vi "Archive Mixed Mode State.vi"(8 "error in":errorcluster, 11 "MixedModeStates":T1) -> (0 "error out":errorcluster, 2 "string":string)   [LabVIEW 2009]
uses:
  Mixed Mode States.ctl
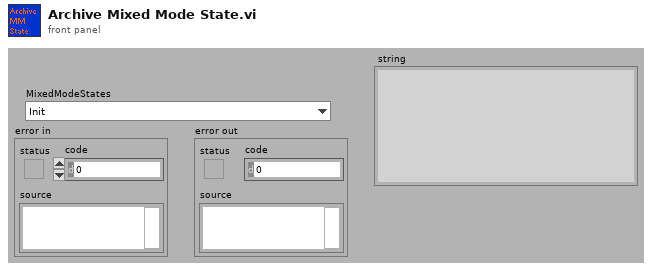
[diagram p1: front panel]
types:
  T1 = typedef "Mixed Mode States.ctl" = enum16{"Init", "Idle", "Start Initial Ramp", "Run Initial Ramp", "Start Iterative Stage", "Convergence Check", "Update Stiffness Jacobian", "Update Command", "Start Iterative Ramp", "Run Iterative Ramp", "Start Iterative Stabilize", "Iterative Stabilize", "Start Iterative Holding", "Iterative Holding", "Start Stabilize", "Stabilize", "Start Hold", "Holding", "Done", "Aborting", "Exit", "Nop"}
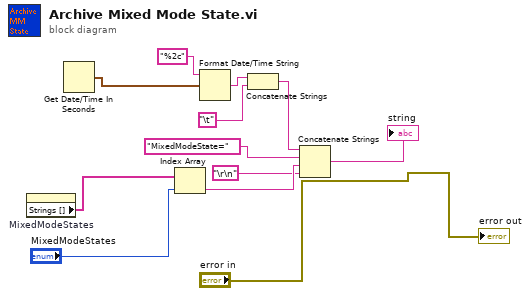
[diagram p0: block diagram]
diagram:
  n1 = property on="MixedModeStates" class="Enum (strict)"() -> ("Strings []"=w12:string[])  [unwired: 2 in, 2 out]
  n2 = Get Date/Time In Seconds() -> (seconds since 1Jan1904=w4:timestamp)
  n3 = Index Array(array=w12, index="MixedModeStates") -> (element=w9:string)
  n4 = Format Date/Time String(time format string (%c)="%2c", seconds (now)=w4) -> (date/time string=w2:string)  [unwired: 1 in]
  n5 = Concatenate Strings(w2, "\t") -> (w3:string)
  n6 = Concatenate Strings(w3, "MixedModeState=" ("string"), w9, "\r\n") -> (→"string":string)
  "error out" <- "error in"
